vi "ExtendedKalmanFilter_GetP_Single.vi"(9 "Col":i32, 10 "Row":i32, 11 "in ExtendedKalmanFiilter":T1) -> (3 "P Pvalue":dbl)   [LabVIEW 2019, in "Trajectory_Library.lvlib"]
doc: "Creates a new LINEAR SYSTEM data cluster with the specified values. \n\n\nInputs: \n - XXX -- XXX.\n\nOutputs:\n - XXX -- XXX."
uses:
  <vilib>/Analysis/Matrix/Datatypes/RealMatrix.ctl
  Trajectory_Library.lvlib
  <vilib>/Analysis/Matrix/NI_Matrix.lvlib
  EXTENDED_KALMAN_FILTER.ctl
panel:
  # "State Estimate <Statess,1>"
  # "<States, States>"
  # "<States, States>"
  # "<Statess,  States>"
  # "<Outputs, Outputs>"
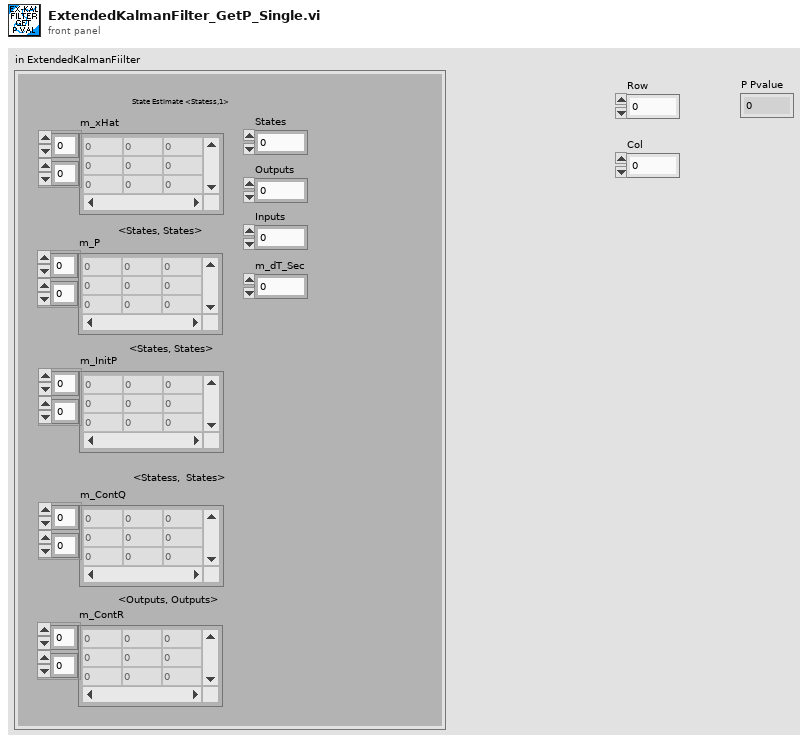
[diagram p1: front panel]
types:
  T1 = typedef "Trajectory_Library.lvlib/EXTENDED_KALMAN_FILTER.ctl" = cluster{"m_P":T2, "m_xHat":T2, "States":i32, "Outputs":i32, "m_ContR":T2, "m_ContQ":T2, "m_dT_Sec":dbl, "Inputs":i32, "m_InitP":T2}
  T2 = typedef "NI_Matrix.lvlib/RealMatrix.ctl" = dbl[][]
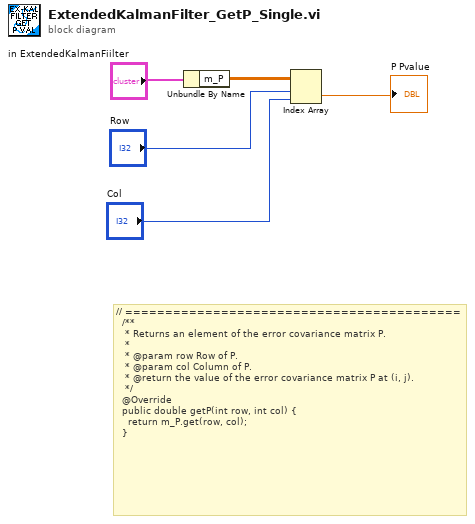
[diagram p0: block diagram]
diagram:
  # "// ==========================================\n  /**\n   * Returns an element of the error covariance matrix P.\n   *\n   * @param row Row of P.\n   * @param col Column of P.\n   * @return the value of the error covariance matrix P at (i, j).\n   */\n  @Override\n  public double getP(int row, int col) {\n    return m_P.get(row, col);\n  }"
  n1 = Unbundle By Name("in ExtendedKalmanFiilter") -> ("m_P"=w4:T2)
  n2 = Index Array(array=w4, index (row)="Row", index (col)="Col") -> (element=→"P Pvalue":dbl)
